vi "GA Home Set Prm Single.vi"(0 "iAxisNum":i16, 1 "dHomeRapidVel":dbl, 2 "dHomeIndexVel":dbl, 5 "nHomeMode":i16, 7 "nHomeDir":i16, 9 "lOffset":i32, 11 "error in (no error)":errorcluster caption="错误输入（无错误）", 12 "dHomeLocatVel":dbl, 13 "dHomeAcc":dbl) -> (4 "function return":i32, 15 "error out":errorcluster caption="错误输出")   [LabVIEW 2015, in "GAS.lvlib"]
doc: "extern \"C\" __declspec(dllimport) int GA_HomeSetPrmSingle(short iAxisNum,short nHomeMode,short nHomeDir,long lOffset,double dHomeRapidVel,double dHomeLocatVel,double dHomeIndexVel,double dHomeAcc);"
uses:
  <userlib>/BP_GAS/GAS.lvlib
  <userlib>/BP_GAS/GAS.dll
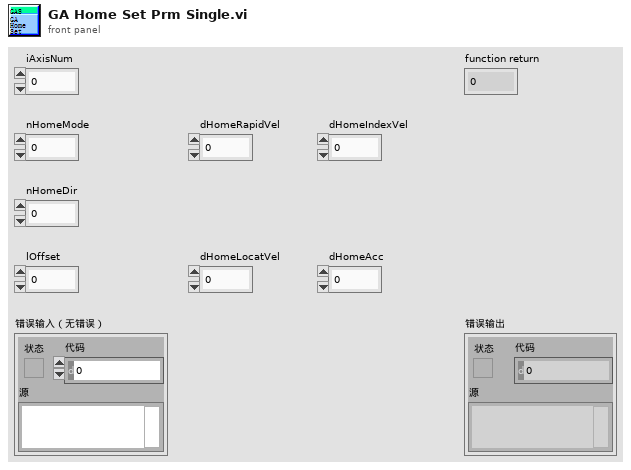
[diagram p1: front panel]
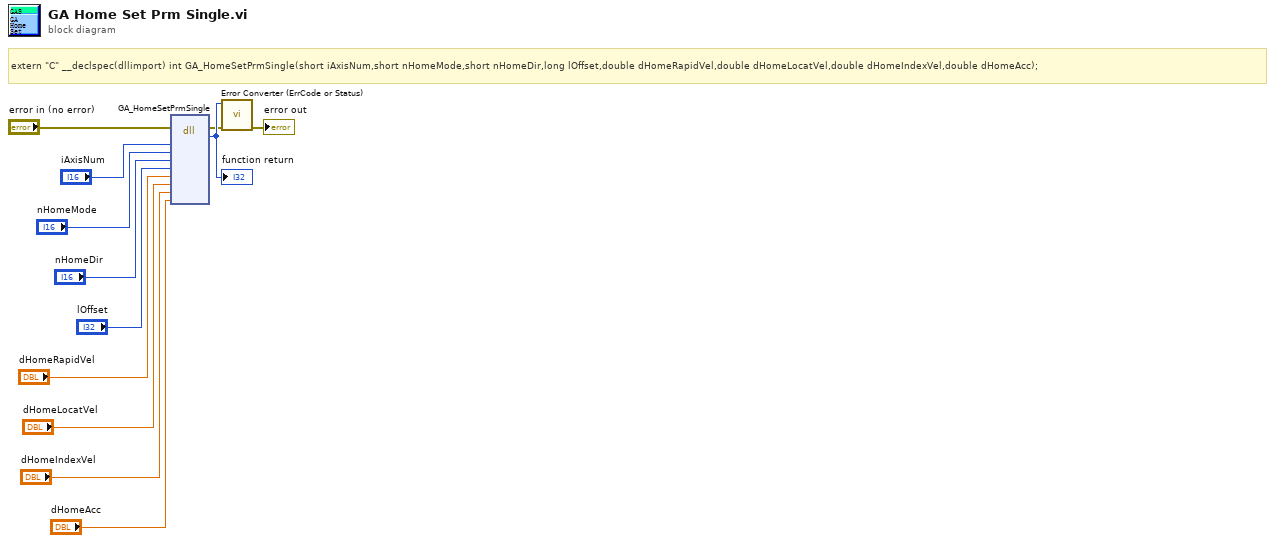
[diagram p0: block diagram]
diagram:
  # "extern \"C\" __declspec(dllimport) int GA_HomeSetPrmSingle(short iAxisNum,short nHomeMode,short nHomeDir,long lOffset,double dHomeRapidVel,double dHomeLocatVel,double dHomeIndexVel,double dHomeAcc);"
  n1 = dll-call lib="E:/Program Files (x86)/National Instruments/LabVIEW 2015/user.lib/BP_GAS/GAS.*" fn="GA_HomeSetPrmSingle"(error in="error in (no error)", "iAxisNum"="iAxisNum", "nHomeMode"="nHomeMode", "nHomeDir"="nHomeDir", "lOffset"="lOffset", "dHomeRapidVel"="dHomeRapidVel", "dHomeLocatVel"="dHomeLocatVel", "dHomeIndexVel"="dHomeIndexVel", "dHomeAcc"="dHomeAcc") -> (error out=w2:errorcluster, w12:i32)  [unwired: 10 in, 1 out]
  "function return" <- w12
  n2 = call "Error Converter (ErrCode or Status).vi"("error in (no error)"=w2, "error code"=w12) -> ("error out"=→"error out":errorcluster)  [unwired: 9 in]
